vi "write_2darray_to_opened_csv.vi"(8 "error in":errorcluster, 9 "Data_in":dbl[][](array[numeric]), 11 "file_ref_in":refnum<file>) -> (0 "error out":errorcluster, 3 "file_ref_out":refnum<file>)   [LabVIEW 2017]
panel:
  out "spreadsheet string":string
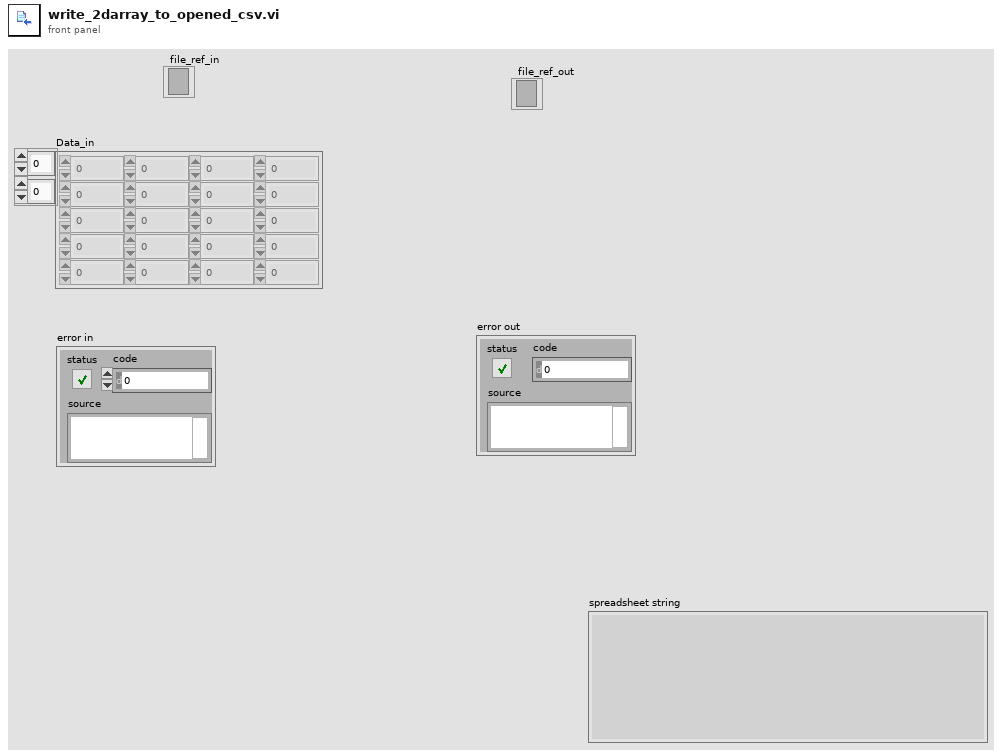
[diagram p1: front panel]
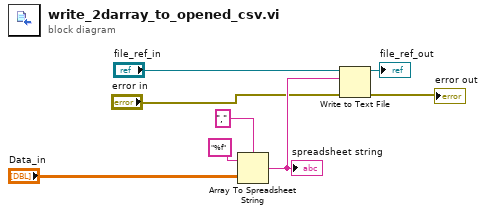
[diagram p0: block diagram]
diagram:
  n1 = Array To Spreadsheet String(delimiter (Tab)=",", array="Data_in", 3:"%f") -> (spreadsheet string=w5:string)
  "spreadsheet string" <- w5
  n2 = Write to Text File(file (use dialog)="file_ref_in", text=w5, error in="error in") -> (refnum out=→"file_ref_out":refnum<file>, error out=→"error out":errorcluster)  [unwired: 1 in, 1 out]
